vi "Write factorPassAlreadyCalculated_.vi"(8 "error in (no error)":errorcluster, 10 "factorPassAlreadyCalculated?":bool, 11 "5RobotsPassGamePlay in":refnum<class "5RobotsPassGamePlay.lvclass">) -> (0 "error out":errorcluster, 3 "5RobotsPassGamePlay out":refnum<class "5RobotsPassGamePlay.lvclass">)   [LabVIEW 2023, in "5RobotsPassGamePlay.lvclass"]
uses:
  5RobotsPassGamePlay.lvclass
  5RobotsPassGamePlay.lvclass/5RobotsPassGamePlay.ctl
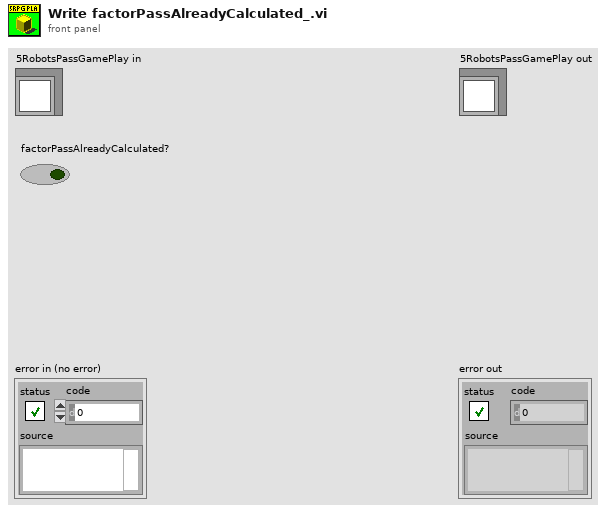
[diagram p1: front panel]
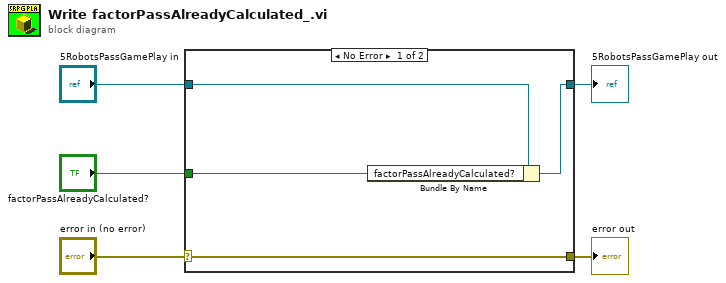
[diagram p0: block diagram]
diagram:
  n1 = case shown="No Error" "error in (no error)" {
    selector: "error in (no error)" -> [w9 w10]
    tunnel: [w9 w10] -> w4
    tunnel: [w7 w11] -> w2
    tunnel: "5RobotsPassGamePlay in" -> [w8 w11]
    tunnel: "factorPassAlreadyCalculated?" -> [w6 _]
    frame No Error {
      n2 = Bundle By Name(cluster=w8, "factorPassAlreadyCalculated?"=w6) -> (w7:refnum<class "5RobotsPassGamePlay.lvclass">)
    }
    frame Error {
    }
  }
  "error out" <- w4
  "5RobotsPassGamePlay out" <- w2
